vi "Read Function (0_ DC Voltage).vi"(8 "error in (no error)":errorcluster, 11 "Agilent_3458 in":refnum<class "Agilent_3458.lvclass">) -> (0 "error out":errorcluster, 2 "Function (0: DC Voltage)":u16(ring) items=["DC Voltage", "AC Voltage", "AC + DC Voltage", "DC Current", "AC Current", "AC + DC Current", "2-Wire Resistance", "4-Wire Resistance", "Frequency", "Period", "Direct Sampling DC", "Direct Sampling AC", "Sub-Sampling DC", "Sub-Sampling AC"], 3 "Agilent_3458 out":refnum<class "Agilent_3458.lvclass">)   [LabVIEW 2018, in "DigitizerPlugins.lvlib" / "Agilent_3458.lvclass"]
uses:
  Agilent_3458.lvclass
  Agilent_3458.lvclass/Agilent_3458.ctl
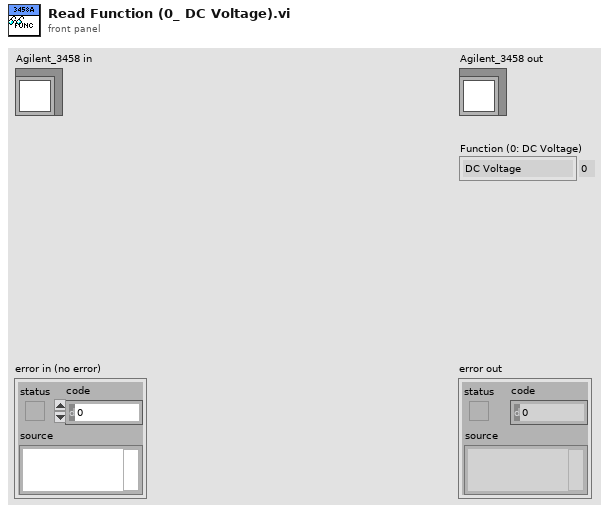
[diagram p1: front panel]
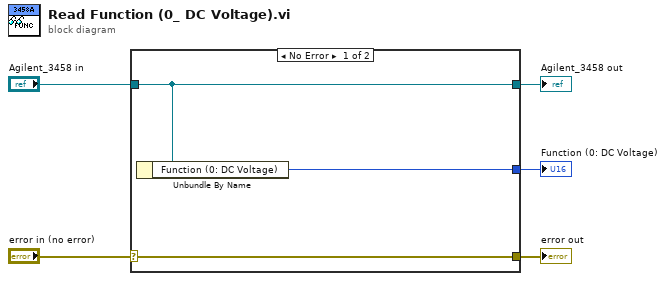
[diagram p0: block diagram]
diagram:
  n1 = case shown="No Error" "error in (no error)" {
    selector: "error in (no error)" -> [w8 w9]
    tunnel: [w8 w9] -> w4
    tunnel: [w7 w10] -> w2
    tunnel: "Agilent_3458 in" -> [w7 w10]
    tunnel: [w6 _] -> w1
    frame No Error {
      n2 = Unbundle By Name(w7) -> ("Function (0: DC Voltage)"=w6:u16)
    }
    frame Error {
    }
  }
  "error out" <- w4
  "Agilent_3458 out" <- w2
  "Function (0: DC Voltage)" <- w1
